vi "UDP dSpace Sender.vi"(6 "ENQUE DIRECTLY":refnum<queue>, 7 "milliseconds to wait":u32, 8 "error in (no error)":errorcluster, 9 "destination adress":string, 10 "destination port":u16, 11 "UDP Network Connection in":refnum<k16>) -> (0 "error out":errorcluster)   [LabVIEW 2016]
uses:
  Globale Variablen VI/Global Variables.vi
  Globale Variablen VI/RadSensoren.vi
  Globale Variablen VI/AutonomousMode.vi
panel:
  out "ss":dbl
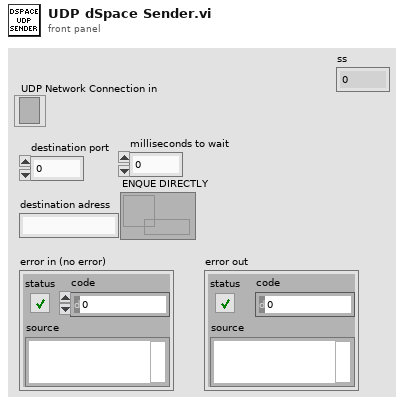
[diagram p1: front panel]
types:
  T1 = enum16{"big-endian, network order", "native, host order", "little-endian"}
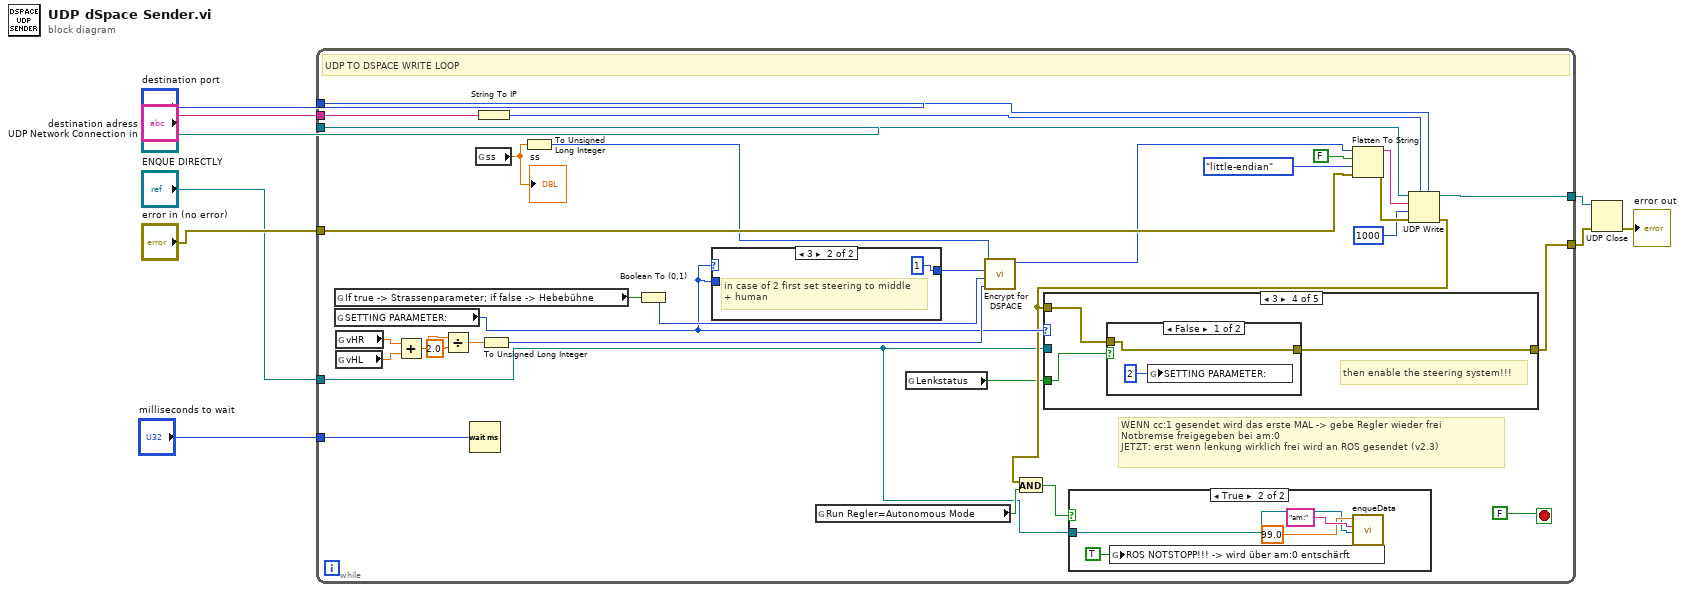
[diagram p0: block diagram]
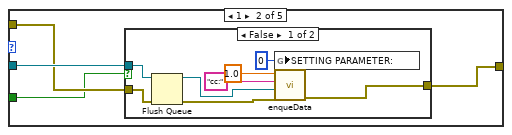
[diagram p5: hidden frame]
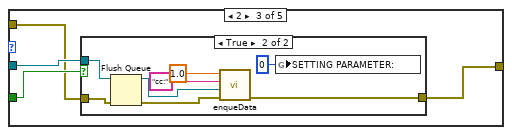
[diagram p7: hidden frame]
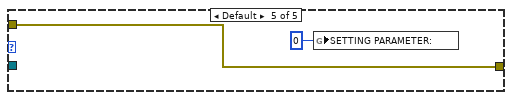
[diagram p10: hidden frame]
diagram:
  n1 = while {
    tunnel: [w22] -> w6
    tunnel: [w41] -> w7
    tunnel: "error in (no error)" -> [w33]
    tunnel: "UDP Network Connection in" -> [w40]
    tunnel: "destination port" -> [w39]
    tunnel: "destination adress" -> [w35]
    tunnel: "milliseconds to wait" -> [w31]
    tunnel: "ENQUE DIRECTLY" -> [w12]
    stop <- FALSE stop-if-true
    # "WENN cc:1 gesendet wird das erste MAL -> gebe Regler wieder frei\nNotbremse freigegeben bei am:0\nJETZT: erst wenn lenkung wirklich frei wird an ROS gesendet (v2.3)"
    # "UDP TO DSPACE WRITE LOOP"
    n2 = global read "AutonomousMode.vi" "If true -> Strassenparameter; if false -> Hebebühne"() -> (w23:bool)
    n3 = global read "Global Variables.vi" "SETTING PARAMETER:"() -> (w17:i32)
    n4 = global read "RadSensoren.vi" "vHR"() -> (w27:sgl)
    n5 = global read "RadSensoren.vi" "vHL"() -> (w28:sgl)
    n6 = Add(x=w27, y=w28) -> (x+y=w26:sgl)
    n7 = Divide(x=w26, y=sgl 2.0) -> (x/y=w24:sgl)
    n8 = Wait (ms)(milliseconds to wait=w31) -> ()  [unwired: 1 out]
    n9 = global read "Global Variables.vi" "ss"() -> (w29:dbl)
    "ss" <- w29
    n10 = String To IP(1:w35) -> (0:w34:u32)
    n11 = To Unsigned Long Integer(number=w24) -> (unsigned 32bit integer=w19:u32)
    n12 = To Unsigned Long Integer(number=w29) -> (unsigned 32bit integer=w21:u32)
    n13 = Boolean To (0,1)(Boolean=w23) -> (0, 1=w20:i16)
    n14 = case shown="3" w17 {
      tunnel: w17 -> [w46 _]
      tunnel: [w46 1] -> w16
      frame Default {
      }
      frame 3 {
        # "in case of 2 first set steering to middle \n+ human"
      }
    }
    n15 = global read "AutonomousMode.vi" "Run Regler=Autonomous Mode"() -> (w15:bool)
    n16 = global read "Global Variables.vi" "Lenkstatus"() -> (w10:bool)
    n17 = call "Encrypt for DSPACE.vi"("ss"=w21, "SETTING PARAMETER:"=w16, "Hebe or Street"=w20, "velocity"=w19) -> ("Message for dSpace"=w18:u32)  [unwired: 6 in]
    n18 = Flatten To String(anything=w18, prepend array or string size? (T)=FALSE, byte order (0:big-endian, network order)=T1."little-endian", error in (no error)=w33) -> (data string=w38:string, error out=w32:errorcluster)  [unwired: 1 out]
    n19 = UDP Write(address=w34, port or service name=w39, connection ID=w40, data in=w38, 8:w32, 9:1000 ("timeout ms (25000)")) -> (error out=w13:errorcluster, 3:w41:refnum<k16>)
    n20 = And(x=w13, y=w15) -> (x .and. y?=w14:bool)
    n21 = case shown="3" w17 {
      tunnel: w13 -> [w48 w50 w63 w76 w81]
      tunnel: w12 -> [_ w52 w64 _ _]
      tunnel: [w48 w51 w62 w75 w81] -> w22
      tunnel: w10 -> [_ w49 w65 w77 _]
      frame 0 {
      }
      frame 1 {
        n22 = case shown="False" w49 {
          tunnel: w52 -> [w59 _]
          tunnel: [w54 w61] -> w51
          tunnel: w50 -> [w53 w61]
          frame False {
            n23 = Flush Queue(queue=w59, error in (no error)=w53) -> (queue out=w56:refnum<queue>, error out=w55:errorcluster)  [unwired: 1 out]
            n24 = global write "Global Variables.vi" "SETTING PARAMETER:"(0 ("SETTING PARAMETER:")) -> ()
            n25 = call "enqueData.vi"("error in (no error)"=w55, "Queue Reference"=w56, "Descriptor"="cc:", "Value IN"=1.0) -> ("error out"=w54:errorcluster)  [unwired: 7 in]
          }
          frame True {
          }
        }
      }
      frame 2 {
        n26 = case shown="True" w65 {
          tunnel: w64 -> [_ w69]
          tunnel: w63 -> [w66 w68]
          tunnel: [w66 w67] -> w62
          frame False {
          }
          frame True {
            n27 = Flush Queue(queue=w69, error in (no error)=w68) -> (queue out=w73:refnum<queue>, error out=w74:errorcluster)  [unwired: 1 out]
            n28 = call "enqueData.vi"("error in (no error)"=w74, "Queue Reference"=w73, "Descriptor"="cc:", "Value IN"=1.0) -> ("error out"=w67:errorcluster)  [unwired: 7 in]
            n29 = global write "Global Variables.vi" "SETTING PARAMETER:"(0 ("SETTING PARAMETER:")) -> ()
          }
        }
      }
      frame 3 {
        # "then enable the steering system!!!"
        n30 = case shown="False" w77 {
          tunnel: w76 -> [w79 w80]
          tunnel: [w79 w80] -> w75
          frame False {
            n31 = global write "Global Variables.vi" "SETTING PARAMETER:"(2 ("SETTING PARAMETER:")) -> ()
          }
          frame True {
          }
        }
      }
      frame Default {
        n32 = global write "Global Variables.vi" "SETTING PARAMETER:"(0 ("SETTING PARAMETER:")) -> ()
      }
    }
    n33 = case shown="True" w14 {
      tunnel: w12 -> [_ w42]
      frame False {
      }
      frame True {
        n34 = global write "AutonomousMode.vi" "ROS NOTSTOPP!!! -> wird über am:0 entschärft"(TRUE ("ROS NOTSTOPP!!! -> wird über am:0 entschärft")) -> ()
        n35 = call "enqueData.vi"("Queue Reference"=w42, "Descriptor"="am:", "Value IN"=99.0) -> ()  [unwired: 8 in, 1 out]
      }
    }
  }
  n36 = UDP Close(connection ID=w7, 8:w6) -> (error out=→"error out":errorcluster)  [unwired: 1 out]
